vi "Apply_Shortcut.vi"(8 "error in (no error)":errorcluster, 9 "shortcut address":T1, 10 "shortcut":refnum<class "IB_Shortcut.lvclass">, 11 "Installer in":refnum<class "Installer.lvclass">) -> (0 "error out":errorcluster, 3 "Installer out":refnum<class "Installer.lvclass">)   [LabVIEW 2020, in "Installer.lvclass"]
uses:
  <vilib>/AppBuilder/IB_Classes/Installer/Installer.lvclass
  <vilib>/AppBuilder/IB_Classes/Installer/Installer.lvclass/Installer.ctl
  <vilib>/AppBuilder/IB_Classes/Source/Container/IB_Source_Container.lvclass
  <vilib>/AppBuilder/IB_Classes/Source/IB_Source.lvclass
  <vilib>/AppBuilder/IB_Classes/Source/File/IB_Source_File.lvclass
  <vilib>/AppBuilder/IB_Classes/Source/File/CtrFile/IB_CtrFile.lvclass
  e:/builds/penguin/labview/branches/2020/dev/dist/vi.lib/AppBuilder/IB_Classes/Source/File/IB_Source_File.lvclass
  e:/builds/penguin/labview/branches/2020/dev/dist/vi.lib/AppBuilder/IB_Classes/Source/IB_Source.lvclass
  e:/builds/penguin/labview/branches/2020/dev/dist/vi.lib/AppBuilder/IB_Classes/Source/File/CtrFile/IB_CtrFile.lvclass
  e:/builds/penguin/labview/branches/2020/dev/dist/vi.lib/AppBuilder/IB_Classes/Source/Container/IB_Source_Container.lvclass
  <vilib>/AppBuilder/IB_Classes/Shortcut/IB_Shortcut.lvclass
  <resource>/Framework/Providers/Builds/Installer/CDK_sTypeDef_ShortcutAddress.ctl
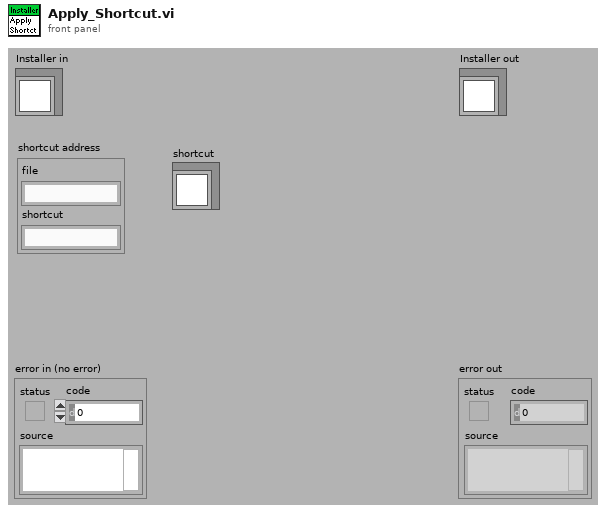
[diagram p1: front panel]
types:
  T1 = typedef "CDK_sTypeDef_ShortcutAddress.ctl" = cluster{"file":string, "shortcut":string}
  T2 = typedef "IB_Source.ctl" = cluster{"name":string, "sourceTag":string, "destTag":string, "path":path, "eng_installPath":string, "UI_inBuild?":bool, "str ref?":bool}
  T3 = typedef "IB_Source_Container.ctl" = cluster{"files":refnum<class "IB_CtrFile.lvclass">[], "previewed?":bool, "preview error?":bool}
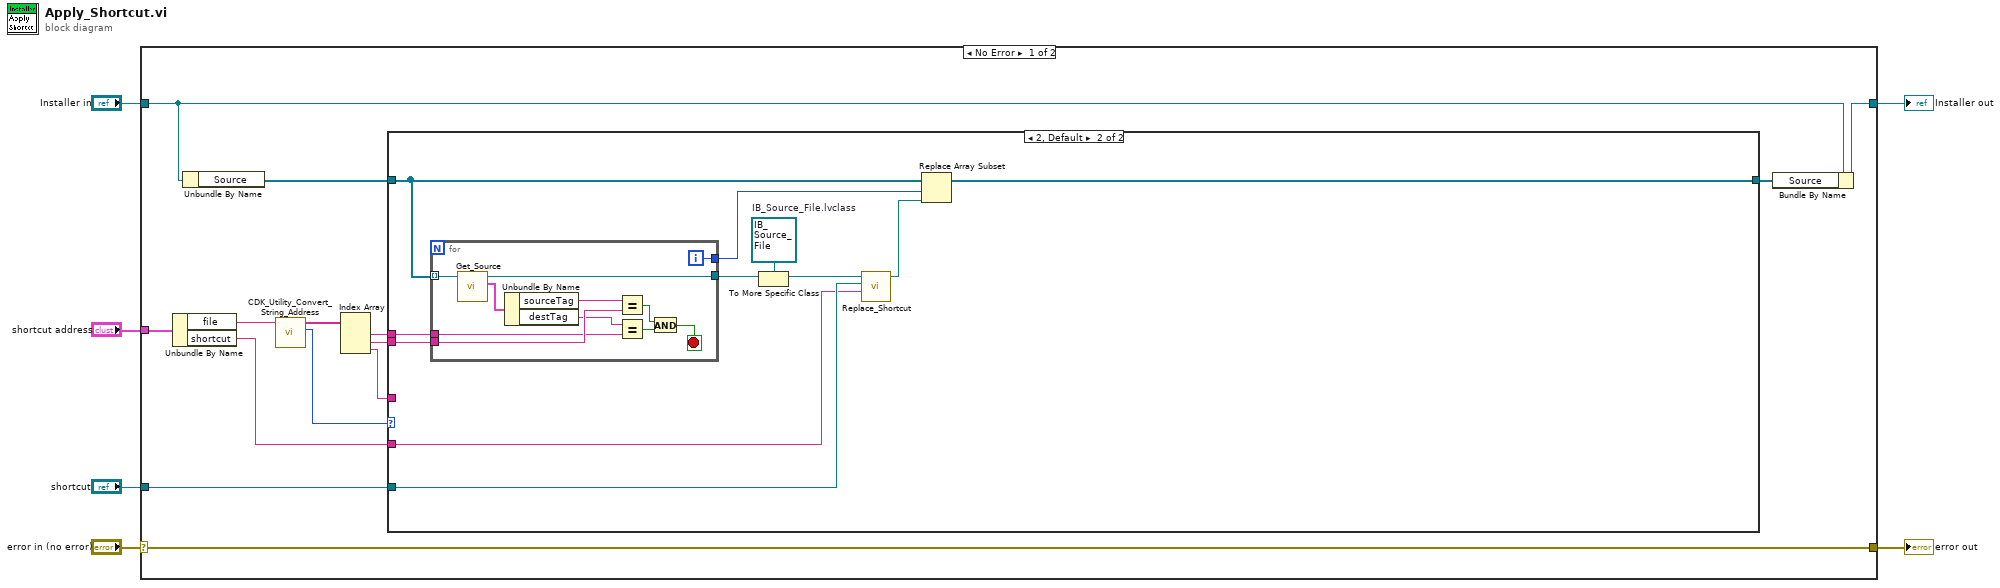
[diagram p0: block diagram]
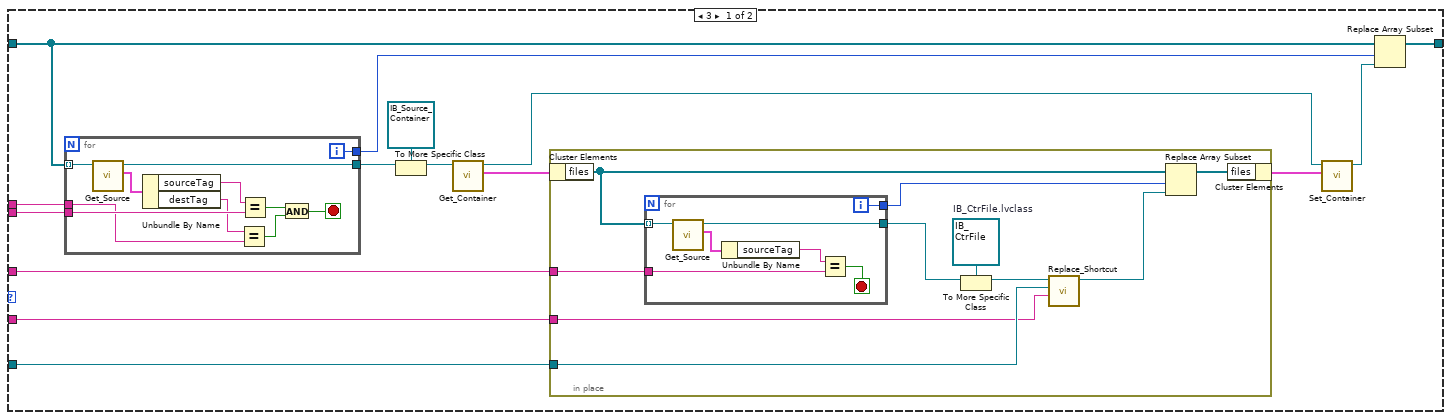
[diagram p2: hidden frame]
diagram:
  n1 = case shown="No Error" "error in (no error)" {
    selector: "error in (no error)" -> [w20 w87]
    tunnel: [w20 w87] -> w4
    tunnel: [w18 w86] -> w3
    tunnel: "Installer in" -> [w19 w86]
    tunnel: "shortcut address" -> [w12 _]
    tunnel: "shortcut" -> [w8 _]
    frame No Error {
      n2 = Unbundle By Name(w12) -> ("file"=w13:string, "shortcut"=w9:string)
      n3 = Unbundle By Name(w19) -> ("Source"=w15:refnum<class "IB_Source.lvclass">[])
      n4 = call <resource>:"CDK_Utility_Convert_String_Address.vi"("address"=w13) -> ("address size"=w10:i32, "address parts"=w11:string[])  [unwired: 9 out]
      n5 = Index Array(array=w11) -> (element #1=w7:string, element #2=w14:string, element #3=w16:string)  [unwired: 3 in]
      n6 = case shown="2, Default" w10 {
        tunnel: [w24 w74] -> w17
        tunnel: w16 -> [w31 _]
        tunnel: w15 -> [w25 w72]
        tunnel: w14 -> [w32 w71]
        tunnel: w9 -> [w22 w65]
        tunnel: w8 -> [w23 w66]
        tunnel: w7 -> [w21 w64]
        frame 3 {
          n7 = for {
            tunnel: w25 -> [w63] mode=indexing
            tunnel: w32 -> [w61]
            tunnel: [w59] -> w33
            tunnel: [w58] -> w26
            tunnel: w21 -> [w56]
            i -> [w58]
            stop <- w55 stop-if-true
            n8 = call <vilib>:"Get_Source.vi"("IB_Source in"=w63) -> ("data"=w60:T2, "IB_Source out"=w59:refnum<class "IB_Source.lvclass">)  [unwired: 1 in, 8 out]
            n9 = Unbundle By Name(w60) -> ("sourceTag"=w62:string, "destTag"=w57:string)
            n10 = Equal?(x=w57, y=w56) -> (x = y?=w53:bool)
            n11 = Equal?(x=w62, y=w61) -> (x = y?=w54:bool)
            n12 = And(x=w54, y=w53) -> (x .and. y?=w55:bool)
          }
          n13 = To More Specific Class(target class=refnum<class "IB_Source_Container.lvclass"> refnum ("IB_Source_Container.lvclass"), reference=w33) -> (specific class reference=w35:refnum<class "IB_Source_Container.lvclass">)  [unwired: 1 in, 1 out]
          n14 = call <vilib>:"Get_Container.vi"("IB_Source_Container in"=w35) -> ("data"=w30:T3, "IB_Source_Container out"=w29:refnum<class "IB_Source_Container.lvclass">)  [unwired: 1 in, 8 out]
          n15 = in-place {
            in-place-border: w31 -> [w45]
            in-place-border: w23 -> [w41]
            in-place-border: w22 -> [w40]
            w39 = refnum<class "IB_CtrFile.lvclass"> refnum  # IB_CtrFile.lvclass
            n16 = in-place-cluster #1(w30) -> ("files"=w43:refnum<class "IB_CtrFile.lvclass">[])
            n17 = for {
              tunnel: w43 -> [w52] mode=indexing
              tunnel: w45 -> [w50]
              tunnel: [w47] -> w44
              tunnel: [w46] -> w37
              i -> [w47]
              stop <- w48 stop-if-true
              n18 = call <vilib>:"Get_Source.vi"("IB_Source in"=w52) -> ("data"=w49:T2, "IB_Source out"=w46:refnum<class "IB_CtrFile.lvclass">)  [unwired: 1 in, 8 out]
              n19 = Unbundle By Name(w49) -> ("sourceTag"=w51:string)
              n20 = Equal?(x=w51, y=w50) -> (x = y?=w48:bool)
            }
            n21 = To More Specific Class(target class=w39, reference=w37) -> (specific class reference=w36:refnum<class "IB_CtrFile.lvclass">)  [unwired: 1 in, 1 out]
            n22 = call <vilib>:"Replace_Shortcut.vi"("shortcut address"=w40, "shortcut"=w41, "IB_Source_File in"=w36) -> ("IB_Source_File out"=w38:refnum<class "IB_CtrFile.lvclass">)  [unwired: 1 in, 7 out]
            n23 = Replace Array Subset(array=w43, new element=w38, index=w44) -> (w42:refnum<class "IB_CtrFile.lvclass">[])
            n24 = in-place-cluster #1("files"=w42) -> (w28:T3)
          }
          n25 = call <vilib>:"Set_Container.vi"("data"=w28, "IB_Source_Container in"=w29) -> ("IB_Source_Container out"=w27:refnum<class "IB_Source_Container.lvclass">)  [unwired: 1 in, 8 out]
          n26 = Replace Array Subset(array=w25, new element=w27, index=w26) -> (w24:refnum<class "IB_Source.lvclass">[])
        }
        frame 2, Default {
          w70 = refnum<class "IB_Source_File.lvclass"> refnum  # IB_Source_File.lvclass
          n27 = for {
            tunnel: w72 -> [w85] mode=indexing
            tunnel: w71 -> [w83]
            tunnel: [w82] -> w73
            tunnel: [w81] -> w69
            tunnel: w64 -> [w78]
            i -> [w82]
            stop <- w75 stop-if-true
            n28 = call <vilib>:"Get_Source.vi"("IB_Source in"=w85) -> ("data"=w80:T2, "IB_Source out"=w81:refnum<class "IB_Source.lvclass">)  [unwired: 1 in, 8 out]
            n29 = Unbundle By Name(w80) -> ("sourceTag"=w84:string, "destTag"=w79:string)
            n30 = Equal?(x=w84, y=w83) -> (x = y?=w77:bool)
            n31 = Equal?(x=w79, y=w78) -> (x = y?=w76:bool)
            n32 = And(x=w77, y=w76) -> (x .and. y?=w75:bool)
          }
          n33 = To More Specific Class(target class=w70, reference=w69) -> (specific class reference=w68:refnum<class "IB_Source_File.lvclass">)  [unwired: 1 in, 1 out]
          n34 = call <vilib>:"Replace_Shortcut.vi"("shortcut address"=w65, "shortcut"=w66, "IB_Source_File in"=w68) -> ("IB_Source_File out"=w67:refnum<class "IB_Source_File.lvclass">)  [unwired: 1 in, 7 out]
          n35 = Replace Array Subset(array=w72, new element=w67, index=w73) -> (w74:refnum<class "IB_Source.lvclass">[])
        }
      }
      n36 = Bundle By Name(cluster=w19, "Source"=w17) -> (w18:refnum<class "Installer.lvclass">)
    }
    frame Error {
    }
  }
  "error out" <- w4
  "Installer out" <- w3
